vi "Frames.Compile.Resp.vi"(8 "error in (no error)":errorcluster, 10 "GUID":string, 11 "Section Ref in":T4 format="%.0x") -> (0 "error out":errorcluster, 2 "Settings":T1 {"Signal.Cmd.Refs"."Signal Refs" format="%.0x"; "Signal.Cmd.Info"."Signals"."Byte Order" items=["Little Endian", "Big Endian"]; "Signal.Cmd.Info"."Signals"."Data Type" items=["Signed", "Unsigned", "IEEE Float"]; "Settings.Refs"."Signal Refs" format="%.0x"; "Signal.Resp.Refs"."Signal Refs" format="%.0x"; "Signal.Resp.Info"."Signals"."Byte Order" items=["Little Endian", "Big Endian"]; "Signal.Resp.Info"."Signals"."Data Type" items=["Signed", "Unsigned", "IEEE Float"]; "Trigger.Refs"."Signal Refs" format="%.0x"; "Status.Refs"."Signal Refs" format="%.0x"}, 3 "Section Ref out":T4 format="%.0x")   [LabVIEW 2019, in "Diagnostics Addon System Explorer.lvlib"]
uses:
  Diagnostics Addon System Explorer.lvlib
  <vilib>/NI VeriStand/Custom Device Tools/Custom Device Utility Library/Custom Device Utility Library.lvlib
  <vilib>/NI VeriStand/Custom Device API/Custom Device API.lvlib
  Types/Frame.Ref.ctl
  Types/FG.Action.ctl
  <vilib>/NI VeriStand/Custom Device API/Custom Device Item Ref.ctl
  Shared/Types/Signal.ctl
  Shared/Diagnostics Addon Shared.lvlib
  Shared/Types/Frame.Compile.ctl
  Shared/Types/Type.ctl
  Types/Service.Export.ctl
  <vilib>/NI VeriStand/Custom Device Tools/Custom Device Utility Library/NI VeriStand - Search for Item by GUID.vi
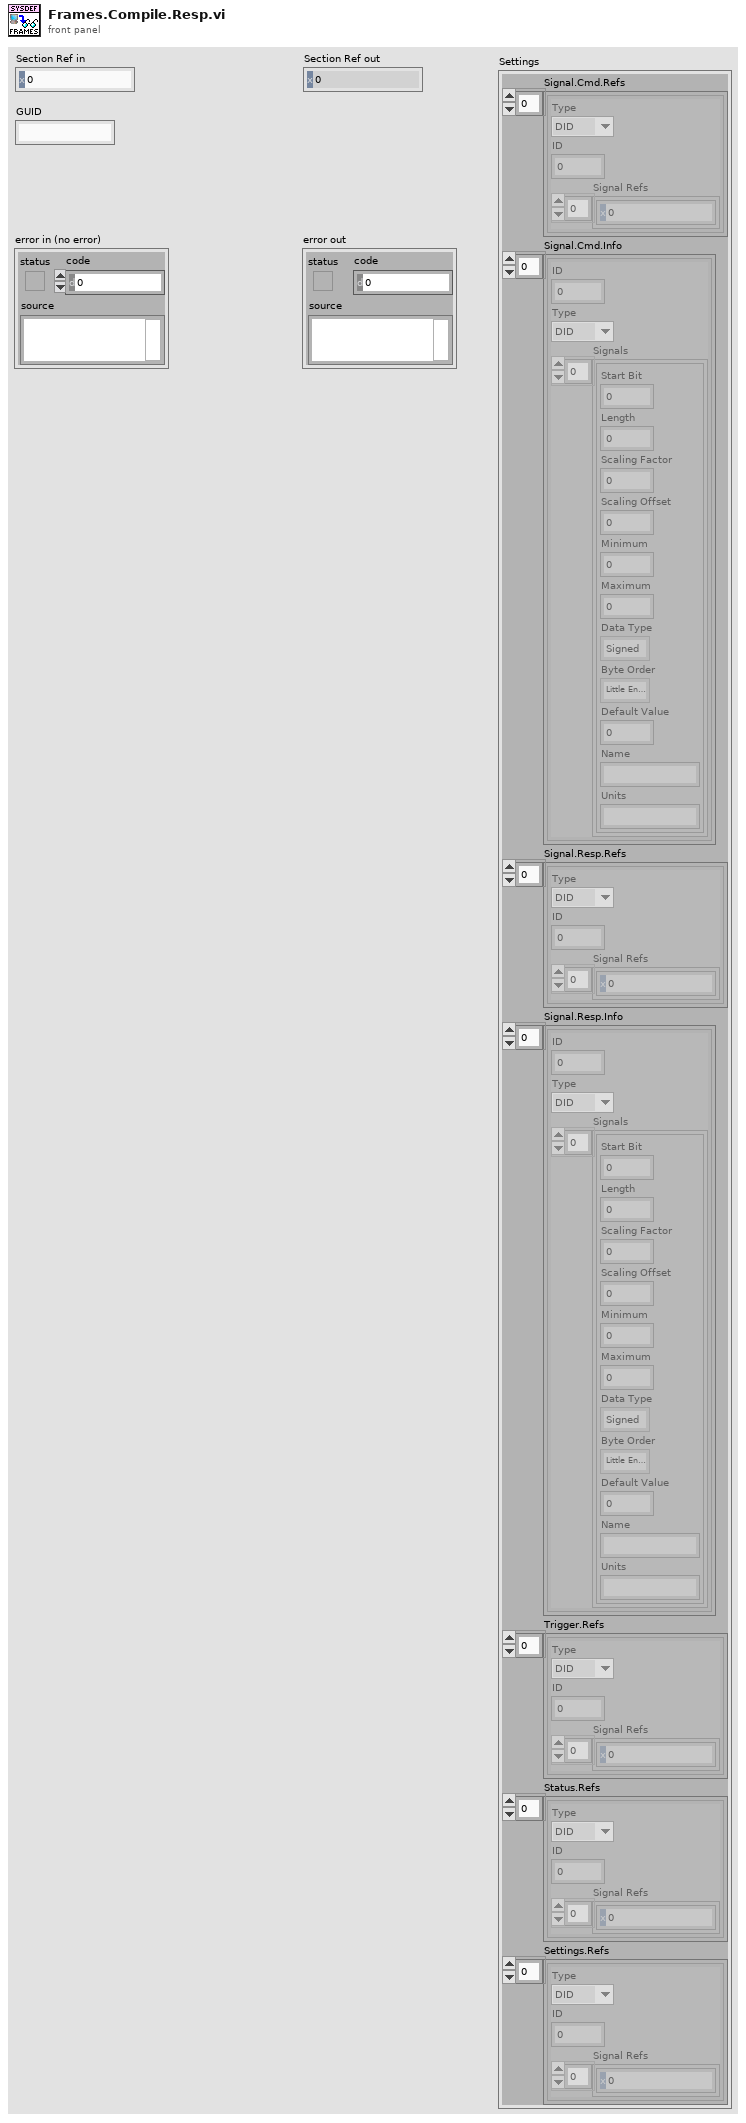
[diagram p1: front panel]
types:
  T1 = typedef "Diagnostics Addon System Explorer.lvlib/Service.Export.ctl" = cluster{"Signal.Cmd.Refs":T2[], "Signal.Cmd.Info":T5[], "Signal.Resp.Refs":T2[], "Signal.Resp.Info":T5[], "Trigger.Refs":T2[], "Status.Refs":T2[], "Settings.Refs":T2[]}
  T2 = typedef "Diagnostics Addon System Explorer.lvlib/Frame.Ref.ctl" = cluster{"Type":T3, "ID":u32, "Signal Refs":T4[]}
  T3 = typedef "Diagnostics Addon Shared.lvlib/Type.ctl" = enum16{"DID", "CDID", "PID", "CPID", "Read Memory", "Write Memory", "IO Control", "Routine Start", "Routine Request", "Routine Stop", "User Defined", "DTC Control", "Clear DTCs", "Read DTCs", "Start DTCs", "DTC Change Count", "Tester Present", "Unlock ECU", "Reset ECU", "Diag Session Control", "Communication Control", "DPID Control", "Poll Control", "Diag CAN Control"}
  T4 = typedef "Custom Device API.lvlib/Custom Device Item Ref.ctl" = u64
  T5 = typedef "Diagnostics Addon Shared.lvlib/Frame.Compile.ctl" = cluster{"ID":u32, "Type":T3, "Signals":T6[]}
  T6 = typedef "Diagnostics Addon Shared.lvlib/Signal.ctl" = cluster{"Start Bit":u32, "Length":u32, "Scaling Factor":dbl, "Scaling Offset":dbl, "Minimum":dbl, "Maximum":dbl, "Data Type":u32, "Byte Order":u32, "Default Value":dbl, "Name":string, "Units":string}
  T7 = typedef "Diagnostics Addon System Explorer.lvlib/FG.Action.ctl" = enum16{"Get", "Set"}
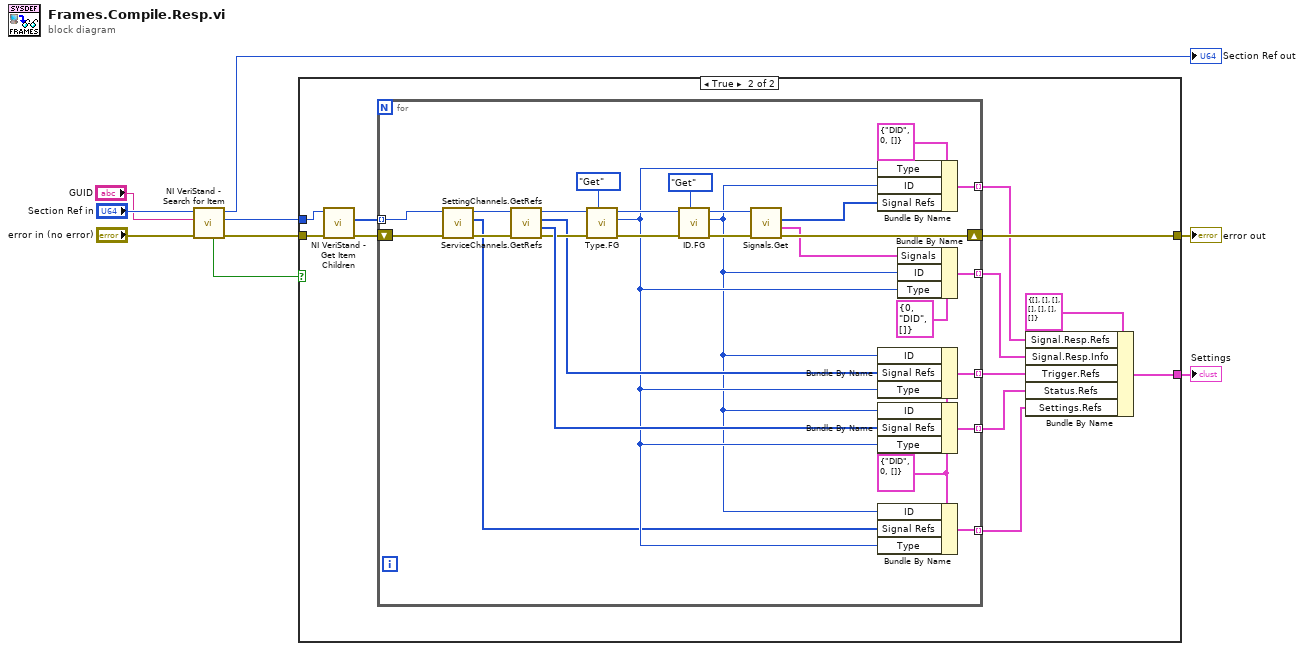
[diagram p0: block diagram]
diagram:
  n1 = call-poly <vilib>:"NI VeriStand - Search for Item.vi"("error in"="error in (no error)", "Item GUID"="GUID", "Section Ref in"="Section Ref in") -> ("error out"=w4:errorcluster, "Item Ref"=w5:T4, "Section Ref out"=→"Section Ref out":T4, "Found"=w2:bool)  [unwired: 5 in]
  n2 = case shown="True" w2 {
    tunnel: [w10 w22] -> w8
    tunnel: w5 -> [_ w19]
    tunnel: w4 -> [w10 w18]
    tunnel: [_ w12] -> w1
    frame False {
    }
    frame True {
      n3 = call <vilib>:"NI VeriStand - Get Item Children.vi"("error in (no error)"=w18, "Item Ref in"=w19) -> ("error out"=w20:errorcluster, "Child Refs"=w21:T4[])  [unwired: 6 in, 2 out]
      n4 = for {
        shift-right: [w45] -> w22
        shift-left: w20 -> [w31]
        tunnel: w21 -> [w28] mode=indexing
        tunnel: [w50] -> w17 mode=indexing
        tunnel: [w42] -> w16 mode=indexing
        tunnel: [w33] -> w15 mode=indexing
        tunnel: [w32] -> w14 mode=indexing
        tunnel: [w23] -> w11 mode=indexing
        w27 = T2 {"Type"=enum."DID", "ID"=0, "Signal Refs"=[]} ("cluster")
        n5 = call "SettingChannels.GetRefs.vi"("error in (no error)"=w31, "Item Ref in"=w28) -> ("error out"=w30:errorcluster, "Settings"=w24:T4[], "Section Ref out"=w29:T4)  [unwired: 7 in]
        n6 = call "ServiceChannels.GetRefs.vi"("error in (no error)"=w30, "Item Ref in"=w29) -> ("error out"=w35:errorcluster, "Status"=w36:T4[], "Trigger"=w34:T4[], "Section Ref out"=w38:T4)  [unwired: 6 in]
        n7 = call "Type.FG.vi"("Action"=FG.Action."Get", "error in (no error)"=w35, "Device Item Ref in"=w38) -> ("error out"=w40:errorcluster, "Type"=w26:T3, "Device Item Ref out"=w41:T4)  [unwired: 6 in]
        n8 = call "ID.FG.vi"("Action"=FG.Action."Get", "error in (no error)"=w40, "Device Item Ref in"=w41) -> ("error out"=w47:errorcluster, "ID"=w25:u32, "Device Item Ref out"=w48:T4)  [unwired: 6 in]
        n9 = call "Signals.Get.vi"("error in (no error)"=w47, "Device Item Ref out"=w48) -> ("error out"=w45:errorcluster, "Parameters"=w43:T6[], "Child Refs"=w46:T4[])  [unwired: 6 in, 1 out]
        n10 = Bundle By Name(cluster=T2 {"Type"=enum."DID", "ID"=0, "Signal Refs"=[]}, "Type"=w26, "ID"=w25, "Signal Refs"=w46) -> (w50:T2)
        n11 = Bundle By Name(cluster=w27, "ID"=w25, "Signal Refs"=w34, "Type"=w26) -> (w33:T2)
        n12 = Bundle By Name(cluster=w27, "ID"=w25, "Signal Refs"=w36, "Type"=w26) -> (w32:T2)
        n13 = Bundle By Name(cluster=w27, "ID"=w25, "Signal Refs"=w24, "Type"=w26) -> (w23:T2)
        n14 = Bundle By Name(cluster=T5 {"ID"=0, "Type"=enum."DID", "Signals"=[]} ("PID In"), "Signals"=w43, "ID"=w25, "Type"=w26) -> (w42:T5)
      }
      n15 = Bundle By Name(cluster=T1 {"Signal.Cmd.Refs"=[], "Signal.Cmd.Info"=[], "Signal.Resp.Refs"=[], "Signal.Resp.Info"=[], "Trigger.Refs"=[], "Status.Refs"=[], "Settings.Refs"=[]}, "Signal.Resp.Refs"=w17, "Signal.Resp.Info"=w16, "Trigger.Refs"=w15, "Status.Refs"=w14, "Settings.Refs"=w11) -> (w12:T1)
    }
  }
  "error out" <- w8
  "Settings" <- w1
